vi "PIEZO_single_write_position.vi"(3 "handle":i32, 4 "error in":errorcluster, 5 "Zposition setpoint":dbl) -> (1 "error out":errorcluster)   [LabVIEW 2015]
uses:
  <userlib>/Madlib.dll
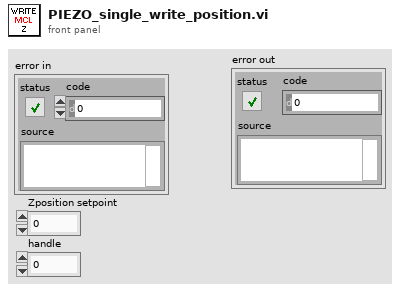
[diagram p1: front panel]
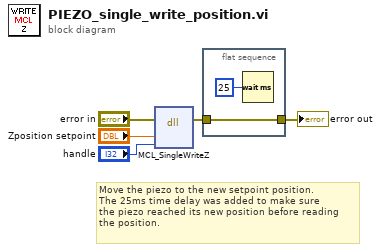
[diagram p0: block diagram]
diagram:
  # "Move the piezo to the new setpoint position.\nThe 25ms time delay was added to make sure \nthe piezo reached its new position before reading\nthe position."
  n1 = dll-call lib="C:/Program Files/National Instruments/LabVIEW 2015/user.lib/Madlib.dll" fn="MCL_SingleWriteZ"(error in="error in", "setpoint"="Zposition setpoint", "handle"="handle") -> (error out=w2:errorcluster)  [unwired: 5 in, 1 out]
  n2 = flat-sequence {
    tunnel: w2 -> [w6]
    tunnel: [w6] -> w1
    frame #0 {
      n3 = Wait (ms)(milliseconds to wait=u32 25) -> ()  [unwired: 1 out]
    }
  }
  "error out" <- w1
